vi "Export to ProjFile VI Entry.vi"(8 "error in (no error)":errorcluster, 11 "LanguageData in":refnum<class "VI Data.lvclass">) -> (0 "error out":errorcluster, 2 "VI Data":T1, 3 "LanguageData out":refnum<class "VI Data.lvclass">)   [LabVIEW 2013, in "SET Project Data.lvlib" / "VI Data.lvclass"]
uses:
  VI Data.lvclass
  Types/ProjFile_VI Data.ctl
  Types/ProjFile_GObject Data.ctl
  VI Data.lvclass/VI Data.ctl
  SET Project Data.lvlib
  Control Classes/GObject/GObject.lvclass
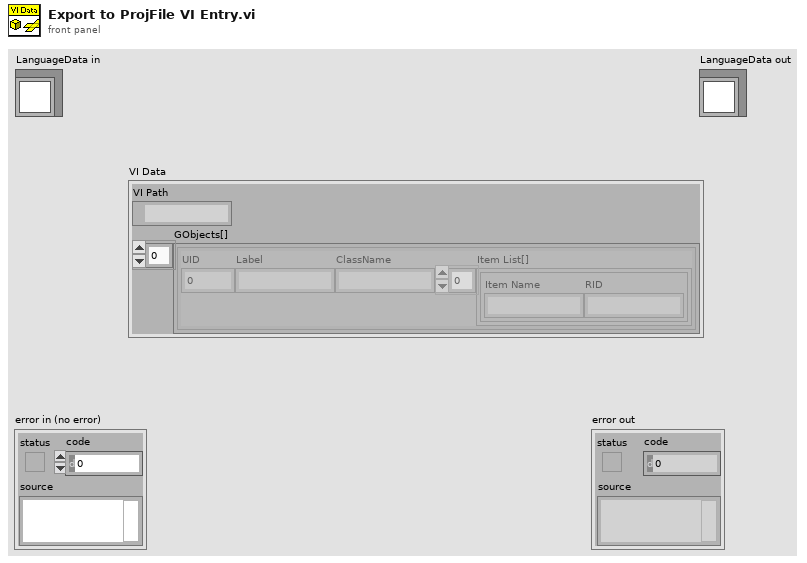
[diagram p1: front panel]
types:
  T1 = typedef "SET Project Data.lvlib/ProjFile_VI Data.ctl" = cluster{"VI Path":path, "GObjects[]":T2[]}
  T2 = typedef "SET Project Data.lvlib/ProjFile_GObject Data.ctl" = cluster{"UID":i32, "Label":string, "ClassName":string, "Item List[]":cluster{"Item Name":string, "RID":string}[]}
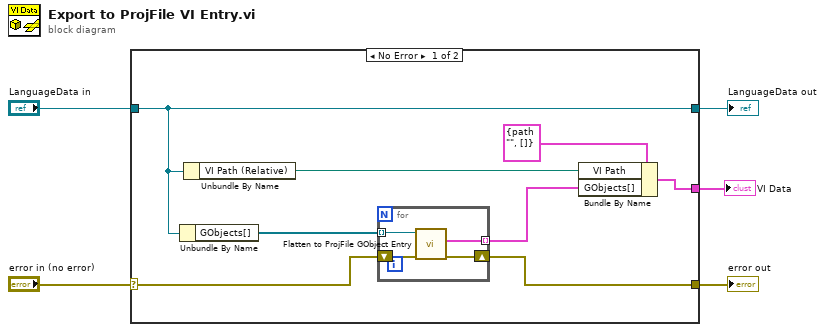
[diagram p0: block diagram]
diagram:
  n1 = case shown="No Error" "error in (no error)" {
    selector: "error in (no error)" -> [w7 w19]
    tunnel: [w6 w19] -> w4
    tunnel: [w13 w18] -> w2
    tunnel: "LanguageData in" -> [w13 w18]
    tunnel: [w10 _] -> w1
    frame No Error {
      n2 = Unbundle By Name(w13) -> ("GObjects[]"=w12:refnum<class "GObject.lvclass">[])
      n3 = Unbundle By Name(w13) -> ("VI Path (Relative)"=w9:path)
      n4 = for {
        tunnel: w12 -> [w17] mode=indexing
        tunnel: [w16] -> w8 mode=indexing
        shift-right: [w14] -> w6
        shift-left: w7 -> [w15]
        n5 = call "Flatten to ProjFile GObject Entry.vi"("error in (no error)"=w15, "GObject in"=w17) -> ("error out"=w14:errorcluster, "GObject Data"=w16:T2)  [unwired: 7 in, 1 out]
      }
      n6 = Bundle By Name(cluster=T1 {"VI Path"=path "", "GObjects[]"=[]} ("VI Data"), "VI Path"=w9, "GObjects[]"=w8) -> (w10:T1)
    }
    frame Error {
    }
  }
  "error out" <- w4
  "LanguageData out" <- w2
  "VI Data" <- w1
